vi "0xE3_Read_one_parameter_of_telemetry_data.vi"(8 "error in":errorcluster, 10 "Номер параметра":i32, 11 "ParamIn":T1={"conParam"={"ReadIntParam"=TRUE, "ReadDescrParam"=FALSE, "ReadFloatParam"=TRUE, "debug"=FALSE, "ReadJSON"=TRUE, "IP_address"="192.168.1.216", "N_attempts"=3, "type_con"=enum."TCP", "MB_address"=1, "VISA"="COM1", "connection ID"=refnum, "nameDevices"="", "timeout"=3000, "port"=2000, "type_version"="0F0C0001", "baud_rate"=115200, "VersionControl"=TRUE, "TCP_conn"=TRUE, "WindowSize"=700}, "Param"={"NumParam"={"NTelem"=201, "NInt"=16, "NFloat"=10, "NTable"=2}, "ParamInt"=[{"ID"="Режим работы", "Num"=0, "Name"="", "Type"="", "Enum"="", "Desc"="", "Unit"="", "Access"="", "FormatStr"="", "Min"=0, "Max"=0}, {"ID"="", "Num"=0, "Name"="", "Type"="", "Enum"="", "Desc"="", "Unit"="", "Access"="", "FormatStr"="", "Min"=0, "Max"=0}, {"ID"="", "Num"=0, "Name"="", "Type"="", "Enum"="", "Desc"="", "Unit"="", "Access"="", "FormatStr"="", "Min"=0, "Max"=0}, {"ID"="", "Num"=0, "Name"="", "Type"="", "Enum"="", "Desc"="", "Unit"="", "Access"="", "FormatStr"="", "Min"=0, "Max"=0}, {"ID"="", "Num"=0, "Name"="", "Type"="", "Enum"="", "Desc"="", "Unit"="", "Access"="", "FormatStr"="", "Min"=0, "Max"=0}, {"ID"="", "Num"=0, "Name"="", "Type"="", "Enum"="", "Desc"="", "Unit"="", "Access"="", "FormatStr"="", "Min"=0, "Max"=0}, {"ID"="ModeWork", "Num"=0, "Name"="", "Type"="", "Enum"="", "Desc"="", "Unit"="", "Access"="", "FormatStr"="", "Min"=0, "Max"=0}], "Telemetry"=[], "Table"=[], "ParamFloat"=[]}}) -> (0 "error out":errorcluster, 1 "float number":sgl, 2 "NParam":i32, 3 "ParamOut":T1={"conParam"={"ReadIntParam"=TRUE, "ReadDescrParam"=FALSE, "ReadFloatParam"=TRUE, "debug"=FALSE, "ReadJSON"=TRUE, "IP_address"="192.168.1.216", "N_attempts"=3, "type_con"=enum."TCP", "MB_address"=1, "VISA"="COM1", "connection ID"=refnum, "nameDevices"="", "timeout"=3000, "port"=2000, "type_version"="0F0C0001", "baud_rate"=115200, "VersionControl"=TRUE, "TCP_conn"=TRUE, "WindowSize"=700}, "Param"={"NumParam"={"NTelem"=201, "NInt"=16, "NFloat"=10, "NTable"=2}, "ParamInt"=[{"ID"="Режим работы", "Num"=0, "Name"="", "Type"="", "Enum"="", "Desc"="", "Unit"="", "Access"="", "FormatStr"="", "Min"=0, "Max"=0}, {"ID"="", "Num"=0, "Name"="", "Type"="", "Enum"="", "Desc"="", "Unit"="", "Access"="", "FormatStr"="", "Min"=0, "Max"=0}, {"ID"="", "Num"=0, "Name"="", "Type"="", "Enum"="", "Desc"="", "Unit"="", "Access"="", "FormatStr"="", "Min"=0, "Max"=0}, {"ID"="", "Num"=0, "Name"="", "Type"="", "Enum"="", "Desc"="", "Unit"="", "Access"="", "FormatStr"="", "Min"=0, "Max"=0}, {"ID"="", "Num"=0, "Name"="", "Type"="", "Enum"="", "Desc"="", "Unit"="", "Access"="", "FormatStr"="", "Min"=0, "Max"=0}, {"ID"="", "Num"=0, "Name"="", "Type"="", "Enum"="", "Desc"="", "Unit"="", "Access"="", "FormatStr"="", "Min"=0, "Max"=0}, {"ID"="ModeWork", "Num"=0, "Name"="", "Type"="", "Enum"="", "Desc"="", "Unit"="", "Access"="", "FormatStr"="", "Min"=0, "Max"=0}], "Telemetry"=[], "Table"=[], "ParamFloat"=[]}})   [LabVIEW 2017, in "LV_Unicorn.lvlib"]
uses:
  LV_Unicorn.lvlib
  Control/unicorn_Param.ctl
  Control/unicorn_conn.ctl
  Control/unicorn_JSON.ctl
  Control/unicorn_ParamInt.ctl
  Control/unicorn_Telemetry.ctl
  Control/unicorn_Table.ctl
  Control/unicorn_ParamFloat.ctl
panel:
  out "String out":string
  out "Ответ":string
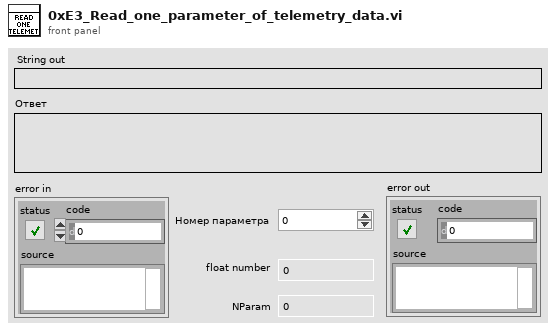
[diagram p1: front panel]
types:
  T1 = typedef "LV_Unicorn.lvlib/unicorn_Param.ctl" = cluster{"conParam":T2, "Param":T3}
  T2 = typedef "LV_Unicorn.lvlib/unicorn_conn.ctl" = cluster{"ReadIntParam":bool, "ReadDescrParam":bool, "ReadFloatParam":bool, "debug":bool, "ReadJSON":bool, "IP_address":string, "N_attempts":i32, "type_con":enum16{"Serial", "TCP"}, "MB_address":i32, "VISA":refnum<visa-resource-name>, "connection ID":refnum<k5>, "nameDevices":string, "timeout":i32, "port":u16, "type_version":string, "baud_rate":u32, "VersionControl":bool, "TCP_conn":bool, "WindowSize":i32}
  T3 = typedef "LV_Unicorn.lvlib/unicorn_JSON.ctl" = cluster{"NumParam":cluster{"NTelem":i32, "NInt":i32, "NFloat":i32, "NTable":i32}, "ParamInt":T4, "Telemetry":T5, "Table":T6, "ParamFloat":T7}
  T4 = typedef "LV_Unicorn.lvlib/unicorn_ParamInt.ctl" = cluster{"ID":string, "Num":i32, "Name":string, "Type":string, "Enum":string, "Desc":string, "Unit":string, "Access":string, "FormatStr":string, "Min":i32, "Max":i32}[]
  T5 = typedef "LV_Unicorn.lvlib/unicorn_Telemetry.ctl" = cluster{"ID":string, "Num":i32, "Name":string, "Desc":string, "Unit":string, "FormatStr":string, "Min":i32, "Max":i32}[]
  T6 = typedef "LV_Unicorn.lvlib/unicorn_Table.ctl" = cluster{"Num":i32, "Access":string, "ColumnCount":i32, "NeedParamPrepare":bool, "Columns":cluster{"Column":i32, "Desc":string, "Name":string}[], "DataType":string, "FormatStr":string, "ID":string, "Name":string, "RowCount":i32, "Rows":cluster{"Desc":string, "ID":string, "Max":i32, "Min":i32, "Name":string, "Row":i32, "Unit":string}[], "Type":string}[]
  T7 = typedef "LV_Unicorn.lvlib/unicorn_ParamFloat.ctl" = cluster{"ID":string, "Num":i32, "Name":string, "Type":string, "Enum":string, "Desc":string, "Unit":string, "Access":string, "FormatStr":string, "Min":sgl, "Max":sgl}[]
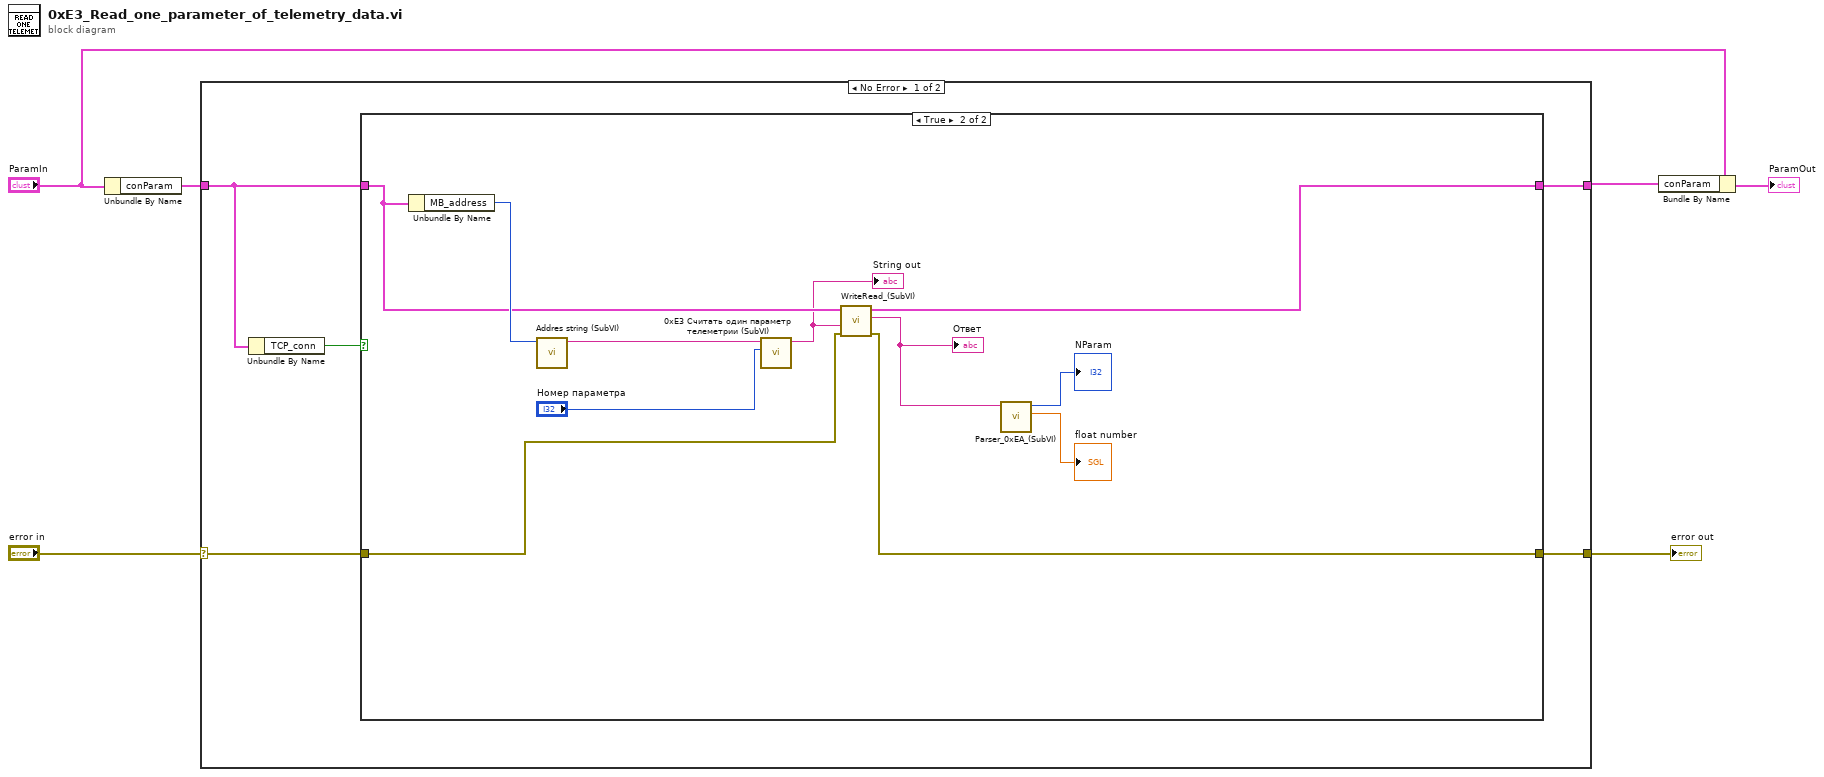
[diagram p0: block diagram]
diagram:
  n1 = Unbundle By Name("ParamIn") -> ("conParam"=w1:T2)
  n2 = case shown="No Error" "error in" {
    selector: "error in" -> [w9 w26]
    tunnel: w1 -> [w8 w25]
    tunnel: [w11 w25] -> w4
    tunnel: [w10 w26] -> w6
    frame No Error {
      n3 = Unbundle By Name(w8) -> ("TCP_conn"=w7:bool)
      n4 = case shown="True" w7 {
        tunnel: [w13 w23] -> w11
        tunnel: [w12 w22] -> w10
        tunnel: w9 -> [w12 w21]
        tunnel: w8 -> [w13 w20]
        frame False {
        }
        frame True {
          n5 = Unbundle By Name(w20) -> ("MB_address"=w24:i32)
          n6 = call "Addres string (SubVI).vi"("Адрес"=w24) -> ("String"=w19:string)  [unwired: 10 in]
          n7 = call "0xE3 Считать один параметр телеметрии (SubVI).vi"("Номер считываемого параметра телеметрии"="Номер параметра", "String in"=w19) -> ("String out"=w17:string)  [unwired: 9 in]
          "String out" <- w17
          n8 = call "WriteRead_(SubVI).vi"("error in"=w21, "Запрос"=w17, "ParamIn"=w20) -> ("error out"=w22:errorcluster, "Ответ"=w16:string, "ParamOut"=w23:T2)  [unwired: 4 in, 2 out]
          "Ответ" <- w16
          n9 = call "Parser_0xEA_(SubVI).vi"("String in"=w16) -> ("float number"=→"float number":sgl, "NParam"=→"NParam":i32)  [unwired: 9 in]
        }
      }
    }
    frame Error {
    }
  }
  "error out" <- w6
  n10 = Bundle By Name(cluster="ParamIn", "conParam"=w4) -> (→"ParamOut":T1)
